vi "PQlistAndCreateColumns.vi"(4 "column type":string, 6 "table":string[](array[string]), 8 "error in":errorcluster, 9 "table name trunc":string, 10 "table name curr":string, 11 "conn":u32) -> (0 "error out":errorcluster, 3 "conn_out":u32)   [LabVIEW 2019, in "libpqutility.lvlib"]
uses:
  libpqutility.lvlib
  PQgetColumn.vi
  libpqlv/src/PQresultErrorMessage.vi
  PQclear.vi
  libpqlv/src/PQsendQuery.vi
  libpqlv/src/PQgetResult.vi
  libpqlv/src/PQresultStatus.vi
  libpqlv/src/PQclear.vi
  PQfetchTables.vi
  libpqlv/src/PQgetvalue.vi
  libpqlv/src/PQntuples.vi
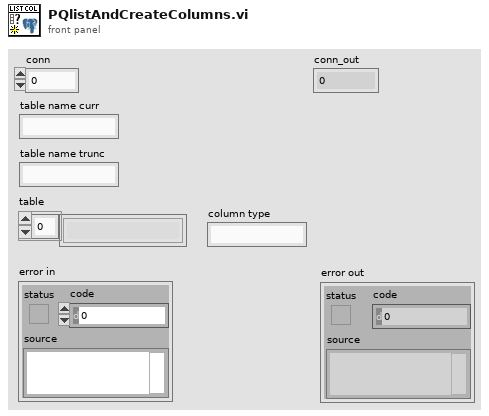
[diagram p1: front panel]
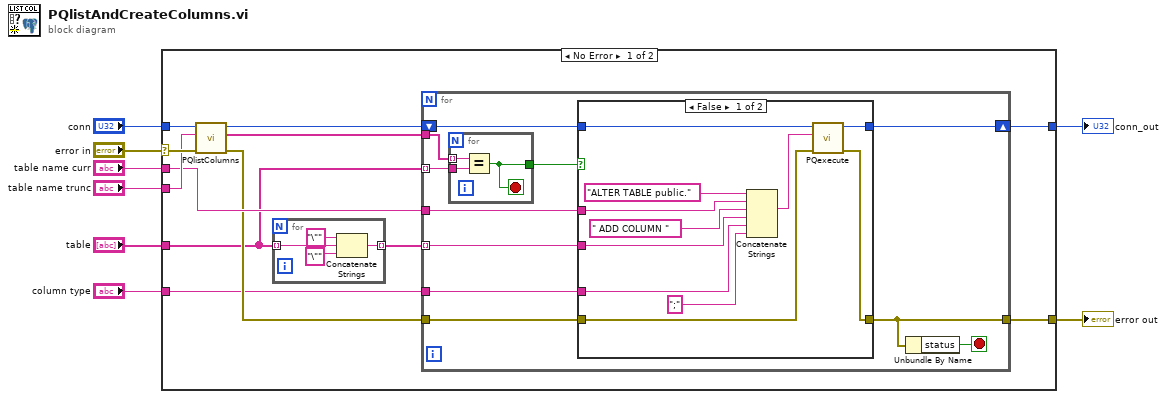
[diagram p0: block diagram]
diagram:
  n1 = case shown="No Error" "error in" {
    selector: "error in" -> [w19 w53]
    tunnel: "conn" -> [w20 w52]
    tunnel: [w9 w52] -> w6
    tunnel: "table" -> [w12 _]
    tunnel: [w13 w53] -> w5
    tunnel: "table name curr" -> [w15 _]
    tunnel: "table name trunc" -> [w17 _]
    tunnel: "column type" -> [w11 _]
    frame No Error {
      n2 = call "PQlistColumns.vi"("error in"=w19, "table"=w17, "conn"=w20) -> ("error out"=w14:errorcluster, "Data"=w16:string[], "conn_out"=w10:u32)  [unwired: 6 in]
      n3 = for {
        tunnel: [w22] -> w18 mode=indexing
        tunnel: w12 -> [w21] mode=indexing
        n4 = Concatenate Strings("\"" ("string"), w21, "\"" ("string")) -> (w22:string)
      }
      n5 = for {
        tunnel: w16 -> [w34]
        tunnel: w12 -> [w35] mode=indexing
        tunnel: w15 -> [w30]
        tunnel: w18 -> [w31] mode=indexing
        tunnel: [w29] -> w13
        tunnel: w14 -> [w27]
        tunnel: w11 -> [w26]
        shift-right: [w25] -> w9
        shift-left: w10 -> [w28]
        stop <- w33 stop-if-true
        n6 = for {
          tunnel: w35 -> [w51]
          tunnel: w34 -> [w50] mode=indexing
          tunnel: [w49] -> w32
          stop <- w49 stop-if-true
          n7 = Equal?(x=w50, y=w51) -> (x = y?=w49:bool)
        }
        n8 = case shown="False" w32 {
          tunnel: w30 -> [w43 _]
          tunnel: w31 -> [w41 _]
          tunnel: [w44 w48] -> w29
          tunnel: w28 -> [w40 w47]
          tunnel: w27 -> [w39 w48]
          tunnel: w26 -> [w37 _]
          tunnel: [w36 w47] -> w25
          frame False {
            n9 = Concatenate Strings("ALTER TABLE public.", w43, " ADD COLUMN ", w41, w37, ";") -> (w45:string)
            n10 = call "PQexecute.vi"("error in"=w39, "SQL querry"=w45, "conn"=w40) -> ("error out"=w44:errorcluster, "conn_out"=w36:u32)  [unwired: 7 in]
          }
          frame True {
          }
        }
        n11 = Unbundle By Name(w29) -> ("status"=w33:bool)
      }
    }
    frame Error {
    }
  }
  "conn_out" <- w6
  "error out" <- w5
